vi "Example Websockets Client-Server.vi"() -> ()   [LabVIEW 2013]
uses:
  Connection/Connection.lvclass
  Connection.Websockets/Connection.WS.lvclass
panel:
  out "Echoed":u8[](array[numeric]) format="%08b"
  out "Sent":u8[](array[numeric]) format="%08b"
  out "server connected":bool
  out "client connected":bool
  out "Comm OK":bool
  out "value":dbl
  out "listener error":errorcluster
  out "client session error":errorcluster
  out "server session error":errorcluster
  out "Received":u8[](array[numeric]) format="%08b"
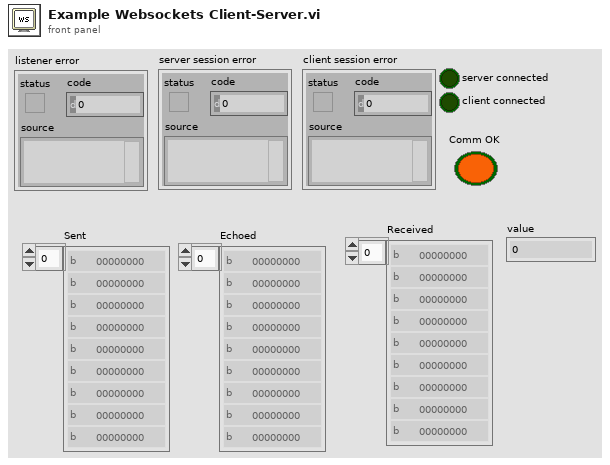
[diagram p1: front panel]
types:
  T1 = typedef "Connection.WS_GOSPL.lvlib/Connection.WS.lvclass/Websocket Frame Type -- ring.ctl" = u8
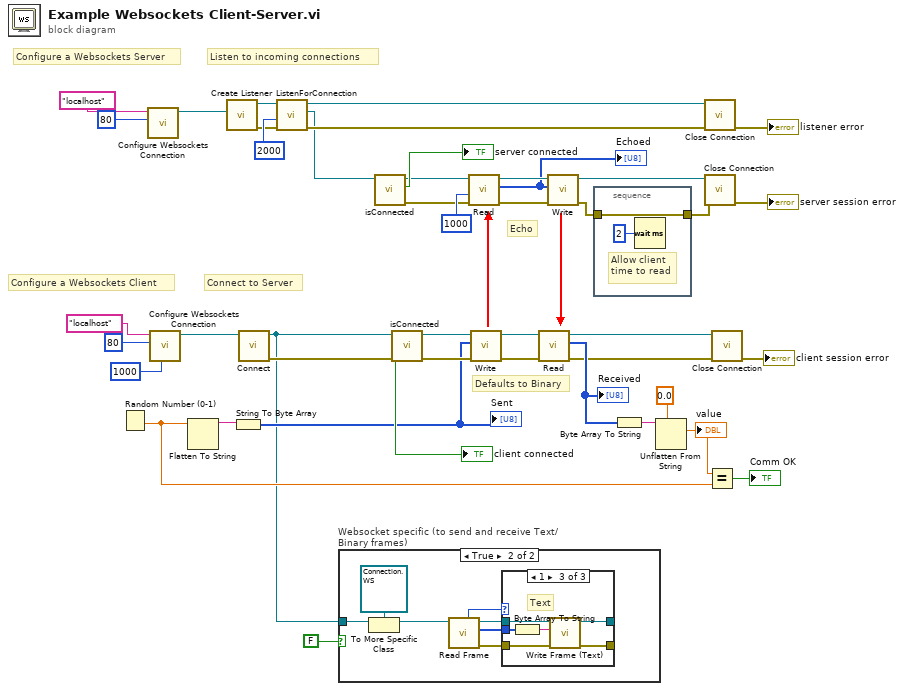
[diagram p0: block diagram]
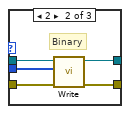
[diagram p4: hidden frame]
diagram:
  # "Defaults to Binary"
  # "Configure a Websockets Client"
  # "Connect to Server"
  # "Echo"
  # "Listen to incoming connections"
  # "Configure a Websockets Server"
  n1 = Random Number (0-1)() -> (number: 0 to 1=w23:dbl)
  n2 = call "Configure Websockets Connection.vi"("remote port (80)"=u16 80, "address (localhost)"="localhost") -> ("Connection.Websockets"=w14:refnum<class "Connection.WS.lvclass">)  [unwired: 8 in, 1 out]
  n3 = call "Configure Websockets Connection.vi"("timeout (5000ms)"=1000, "remote port (80)"=u16 80, "address (localhost)"="localhost") -> ("Connection.Websockets"=w13:refnum<class "Connection.WS.lvclass">)  [unwired: 7 in, 1 out]
  n4 = Flatten To String(anything=w23) -> (data string=w33:string)  [unwired: 3 in, 2 out]
  n5 = call "Create Listener.vi"("Connection Configuration"=w14) -> ("error out"=w41:errorcluster, "Listener"=w44:refnum<class "Connection.WS.lvclass">)  [unwired: 9 in]
  n6 = String To Byte Array(string=w33) -> (unsigned byte array=w5:u8[])
  "Sent" <- w5
  n7 = call "Connect.vi"("Connection in"=w13) -> ("error out"=w3:errorcluster, "Connection out"=w1:refnum<class "Connection.WS.lvclass">)  [unwired: 9 in]
  n8 = call "ListenForConnection.vi"("error in (no error)"=w41, "timeout (2000 ms)"=2000 ("bytes to read (100)"), "Listener"=w44) -> ("error out"=w28:errorcluster, "Connection"=w2:refnum<class "Connection.lvclass">, "Listener out"=w42:refnum<class "Connection.WS.lvclass">)  [unwired: 5 in, 1 out]
  n9 = case "Websocket specific (to send and receive Text/Binary frames)" shown="True" FALSE {
    tunnel: w1 -> [_ w45]
    frame False {
    }
    frame True {
      n10 = To More Specific Class(target class=refnum<class "Connection.WS.lvclass"> refnum ("Connection.WS"), reference=w45) -> (specific class reference=w46:refnum<class "Connection.WS.lvclass">)  [unwired: 1 in, 1 out]
      n11 = call "Read Frame.vi"("Connection.WS"=w46) -> ("error out"=w49:errorcluster, "Bytes"=w50:u8[], "Connection.WS"=w51:refnum<class "Connection.WS.lvclass">, "Frame Type"=w48:T1)  [unwired: 5 in, 2 out]
      n12 = case shown="1" w48 {
        tunnel: [w53 w58 w63] -> _
        tunnel: [w52 w57 w62] -> _
        tunnel: w51 -> [w53 w56 w64]
        tunnel: w50 -> [_ w55 w60]
        tunnel: w49 -> [w52 w54 w61]
        frame Default {
        }
        frame 2 {
          # "Binary"
          n13 = call "Write.vi"("error in (no error)"=w54, "Bytes"=w55, "Connection in"=w56) -> ("error out"=w57:errorcluster, "Connection"=w58:refnum<class "Connection.WS.lvclass">)  [unwired: 7 in]
        }
        frame 1 {
          # "Text"
          n14 = Byte Array To String(unsigned byte array=w60) -> (string=w59:string)
          n15 = call "Write Frame (Text).vi"("error in (no error)"=w61, "Text"=w59, "Connection.WS"=w64) -> ("error out"=w62:errorcluster, "Connection.WS"=w63:refnum<class "Connection.WS.lvclass">)  [unwired: 7 in]
        }
      }
    }
  }
  n16 = call "isConnected.vi"("Connection in"=w2) -> ("error out"=w9:errorcluster, "connected"=→"server connected":bool, "Connection out"=w4:refnum<class "Connection.lvclass">)  [unwired: 8 in]
  n17 = call "isConnected.vi"("error in (no error)"=w3, "Connection in"=w1) -> ("error out"=w8:errorcluster, "connected"=→"client connected":bool, "Connection out"=w18:refnum<class "Connection.WS.lvclass">)  [unwired: 7 in]
  n18 = call "Read.vi"("error in (no error)"=w9, "timeout (2000 ms)"=1000 ("bytes to read (100)"), "TCPConnection in"=w4) -> ("error out"=w37:errorcluster, "Bytes"=w6:u8[], "TCPConnection out"=w39:refnum<class "Connection.lvclass">)  [unwired: 4 in, 2 out]
  "Echoed" <- w6
  n19 = call "Write.vi"("error in (no error)"=w8, "Bytes"=w5, "Connection in"=w18) -> ("error out"=w36:errorcluster, "Connection"=w38:refnum<class "Connection.WS.lvclass">)  [unwired: 7 in]
  n20 = call "Read.vi"("error in (no error)"=w36, "TCPConnection in"=w38) -> ("error out"=w26:errorcluster, "Bytes"=w32:u8[], "TCPConnection out"=w25:refnum<class "Connection.WS.lvclass">)  [unwired: 5 in, 2 out]
  "Received" <- w32
  n21 = call "Write.vi"("error in (no error)"=w37, "Bytes"=w6, "Connection in"=w39) -> ("error out"=w21:errorcluster, "Connection"=w34:refnum<class "Connection.lvclass">)  [unwired: 7 in]
  n22 = stacked-sequence {
    tunnel: w21 -> [w65]
    tunnel: [w65] -> w20
    frame #0 {
      # "Allow client\ntime to read"
      n23 = Wait (ms)(milliseconds to wait=u32 2) -> ()  [unwired: 1 out]
    }
  }
  n24 = Byte Array To String(unsigned byte array=w32) -> (string=w31:string)
  n25 = Unflatten From String(type=0.0, binary string=w31) -> (value=w24:dbl)  [unwired: 3 in, 2 out]
  "value" <- w24
  n26 = call "Close Connection.vi"("error in (no error)"=w28, "Connection in"=w42) -> ("error out"=→"listener error":errorcluster)  [unwired: 8 in, 1 out]
  n27 = call "Close Connection.vi"("error in (no error)"=w20, "Connection in"=w34) -> ("error out"=→"server session error":errorcluster)  [unwired: 8 in, 1 out]
  n28 = Equal?(x=w24, y=w23) -> (x = y?=→"Comm OK":bool)
  n29 = call "Close Connection.vi"("error in (no error)"=w26, "Connection in"=w25) -> ("error out"=→"client session error":errorcluster)  [unwired: 8 in, 1 out]
